vi "test-diff-drive-odom.vi"() -> ()   [LabVIEW 2019]
panel:
  out "T0 -- Ras/sec -- 0":dbl
  out "T0 -- y -- 0":dbl
  out "T0 -- X -- 0":dbl
  # "Diff Drive Odometry Test"
  # "diff Drive Odom is different.... Only implemented Update.....\nThis one is very LabVIEW centric....."
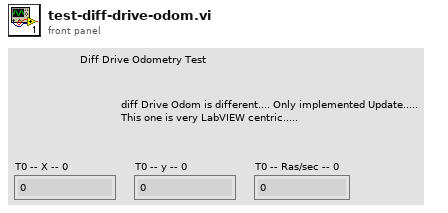
[diagram p1: front panel]
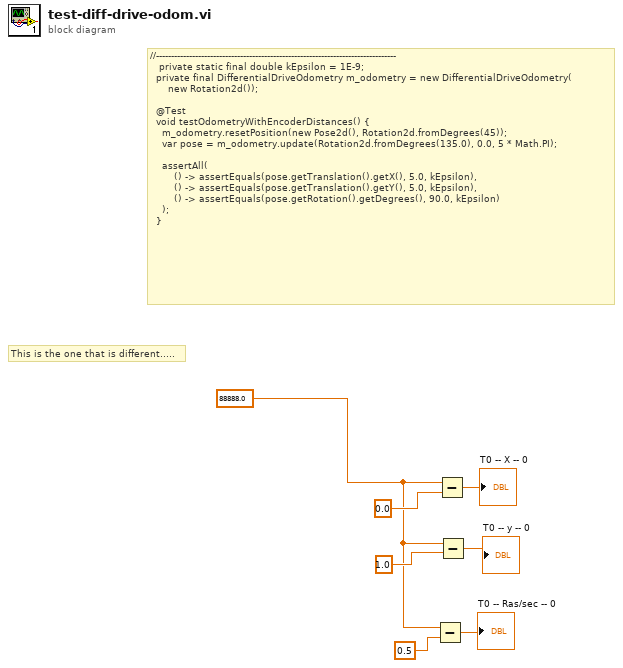
[diagram p0: block diagram]
diagram:
  w1 = 88888.0 ("x")
  # "This is the one that is different....."
  # "//--------------------------------------------------------------------------------\n   private static final double kEpsilon = 1E-9;\n  private final DifferentialDriveOdometry m_odometry = new DifferentialDriveOdometry(\n      new Rotation2d());\n\n  @Test\n  void testOdometryWithEncoderDistances() {\n    m_odometry.resetPosition(new Pose2d(), Rotation2d.fromDegrees(45));\n    var pose = m_odometry.update(Rotation2d.fromDegrees(135.0), 0.0, 5 * Math.PI);\n\n    assertAll(\n        () -> assertEquals(pose.getTranslation().getX(), 5.0, kEpsilon),\n        () -> assertEquals(pose.getTranslation().getY(), 5.0, kEpsilon),\n        () -> assertEquals(pose.getRotation().getDegrees(), 90.0, kEpsilon)\n    );\n  }"
  n1 = Subtract(x=w1, y=0.5) -> (x-y=→"T0 -- Ras/sec -- 0":dbl)
  n2 = Subtract(x=w1, y=0.0) -> (x-y=→"T0 -- X -- 0":dbl)
  n3 = Subtract(x=w1, y=1.0) -> (x-y=→"T0 -- y -- 0":dbl)
